vi "AO-Volt.vi"(6 "Slot":T1, 8 "error in":errorcluster, 10 "Value":string, 11 "CH":string) -> (0 "error out":errorcluster)   [LabVIEW 2013]
uses:
  SystemCode/SysControl/Slot.ctl
  <vilib>/DAQmx/write.llb/DAQmx Write (Analog DBL 1Chan 1Samp).vi
  SourceCode/GlobalValue.vi
  <vilib>/DAQmx/create/channels.llb/DAQmx Create Channel (AO-Voltage-Basic).vi
  <vilib>/DAQmx/miscellaneous.llb/DAQmx Fill In Error Info.vi
panel:
  in  "Operate":enum16{"Set", "Initialize"}(ring)
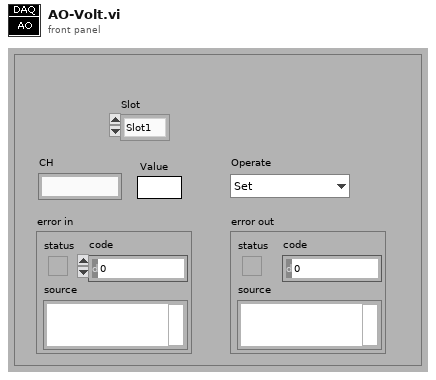
[diagram p1: front panel]
types:
  T1 = typedef "Slot.ctl" = enum16{"Slot1", "Slot2", "Slot3", "Slot4"}
  T2 = typedef "DAQConfig.ctl" = cluster{"DIO":string[][], "AO":string[][], "AI":string[][]}
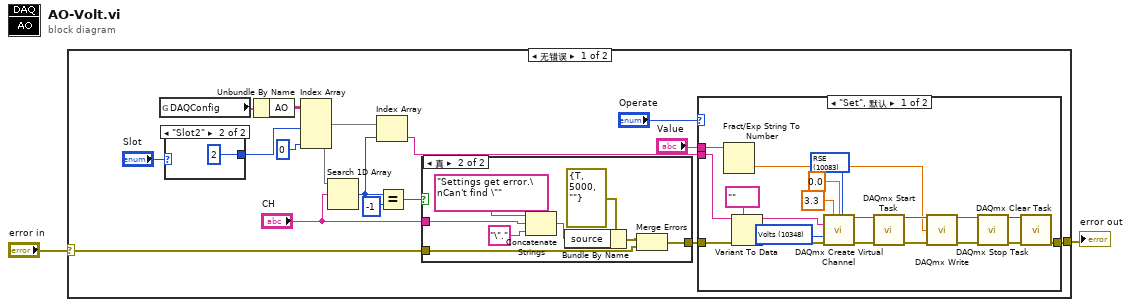
[diagram p0: block diagram]
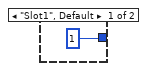
[diagram p2: hidden frame]
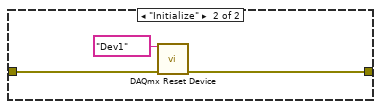
[diagram p4: hidden frame]
diagram:
  n1 = case shown="无错误" "error in" {
    selector: "error in" -> [w6 w54]
    tunnel: [w18 w54] -> w2
    frame No Error {
      n2 = global read "GlobalValue.vi" "DAQConfig"() -> (w3:T2)
      n3 = case shown="\"Slot2\"" "Slot" {
        tunnel: [1 ("索引 (行)") 2 ("索引 (行)")] -> w4
        frame "Slot1", Default {
        }
        frame "Slot2" {
        }
      }
      n4 = Unbundle By Name(w3) -> ("AO"=w16:string[][])
      n5 = Index Array(array=w16, index (col) #1=w4, index (col) #2=0 ("索引 (列)")) -> (element #1=w12:string[], element #2=w11:string[])  [unwired: 2 in]
      n6 = Search 1D Array(1D array=w11, element="CH") -> (index of element=w14:i32)  [unwired: 1 in]
      n7 = Index Array(array=w12, index=w14) -> (element=w8:string)
      n8 = Equal?(x=w14, y=-1) -> (x = y?=w10:bool)
      n9 = case shown="真" w10 {
        tunnel: w6 -> [w22 w26]
        tunnel: [w22 w25] -> w17
        tunnel: "CH" -> [_ w24]
        frame False {
        }
        frame True {
          n10 = Concatenate Strings("Settings get error.\nCan't find \"" ("message"), w24, "\"." ("string")) -> (w29:string)
          n11 = Bundle By Name(cluster=errorcluster {"status"=TRUE, "code"=5000, "source"=""} ("error in 1 (no error)"), "source"=w29) -> (w28:errorcluster)
          n12 = Merge Errors(w28, w26) -> (w25:errorcluster)
        }
      }
      n13 = case shown="\"Set\", 默认" "Operate" {
        tunnel: w17 -> [w34 w53]
        tunnel: [w46 w52] -> w18
        tunnel: w8 -> [w33 _]
        tunnel: "Value" -> [w32 _]
        frame "Set", Default {
          w36 = 10083 items=["Default"=-1, "RSE"=10083, "Differential"=10106, "Pseudodifferential"=12529] ("output terminal configuration")
          w42 = 10348 items=["Volts"=10348, "From Custom Scale"=10065] ("units")
          n14 = Fract/Exp String To Number(string=w32) -> (number=w35:dbl)  [unwired: 3 in, 1 out]
          n15 = Variant To Data(error in=w34, type=tag "" ("lines"), Variant=w33) -> (data=w37:tag, error out=w31:errorcluster)
          n16 = call-poly <vilib>:"DAQmx Create Virtual Channel.vi"("maximum value"=3.3, "minimum value"=0.0, "output terminal configuration"=w36, "physical channels"=w37, "units"=w42, "error in"=w31) -> ("task out"=w38:refnum<k21>, "error out"=w39:errorcluster)  [unwired: 8 in]
          n17 = call <vilib>:"DAQmx Start Task.vi"("task/channels in"=w38, "error in"=w39) -> ("task out"=w50:refnum<k21>, "error out"=w49:errorcluster)  [unwired: 12 in]
          n18 = call-poly <vilib>:"DAQmx Write.vi"("task/channels in"=w50, "data"=w35, "error in"=w49) -> ("task out"=w44:refnum<k21>, "error out"=w43:errorcluster)  [unwired: 10 in, 1 out]
          n19 = call <vilib>:"DAQmx Stop Task.vi"("task/channels in"=w44, "error in"=w43) -> ("task out"=w48:refnum<k21>, "error out"=w47:errorcluster)  [unwired: 12 in]
          n20 = call <vilib>:"DAQmx Clear Task.vi"("task in"=w48, "error in"=w47) -> ("error out"=w46:errorcluster)  [unwired: 13 in]
        }
        frame "Initialize" {
          n21 = call <vilib>:"DAQmx Reset Device.vi"("device in"=tag "Dev1", "error in"=w53) -> ("error out"=w52:errorcluster)  [unwired: 13 in]
        }
      }
    }
    frame Error {
    }
  }
  "error out" <- w2
